vi "Self-Test.vi"(8 "error in (no error)":errorcluster, 11 "VISA resource name":refnum<visa-resource-name>) -> (0 "error out":errorcluster, 1 "Self-Test Response":string, 2 "Self-Test Error":u32, 3 "VISA resource name out":refnum<visa-resource-name>)   [LabVIEW 2015, in "Lake Shore 372.lvlib"]
doc: "Causes the instrument to perform a self-test and returns the results. A numeric indicator indicates if the instrument passed all self-tests, and a string indicator contains the instrument's reponse."
uses:
  <instrlib>/Lake Shore 372/Lake Shore 372.lvlib
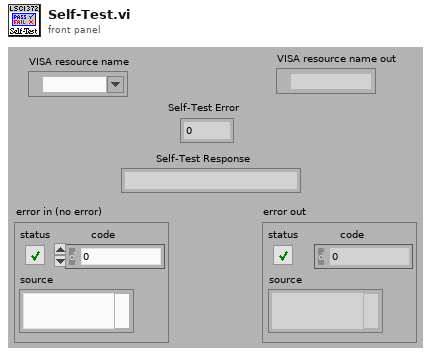
[diagram p1: front panel]
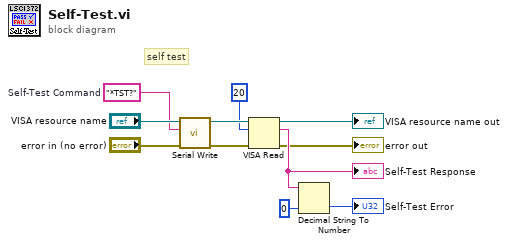
[diagram p0: block diagram]
diagram:
  w2 = "*TST?"  # Self-Test Command
  # "self test"
  n1 = call <instrlib>:"Serial Write.vi"("error in (no error)"="error in (no error)", "Write Buffer (\"\")"=w2, "VISA resource name"="VISA resource name") -> ("error out"=w3:errorcluster, "VISA resource name out"=w5:refnum<visa-resource-name>)  [unwired: 6 in, 1 out]
  n2 = VISA Read(VISA resource name=w5, byte count=u32 20, error in (no error)=w3) -> (VISA resource name out=→"VISA resource name out":refnum<visa-resource-name>, read buffer=w11:string, error out=→"error out":errorcluster)  [unwired: 1 out]
  "Self-Test Response" <- w11
  n3 = Decimal String To Number(string=w11, default (0L)=u32 0 ("Default (0L)")) -> (number=→"Self-Test Error":u32)  [unwired: 1 in, 1 out]
